vi "Configure DO Alarm.vi"(0 "VISA resource name":refnum<visa-resource-name>, 1 "Operation (0: And)":i32(ring) items=["And", "Or", "Reflash"], 2 "Hold / Non-Hold (Non-Hold)":bool, 3 "Operation When ACK (Normal)":u16(ring) items=["Normal", "Reset"], 5 "Channel Number (0001)":string="0001", 7 "Span And Energize":T1={"Span Lower Limit (0)"=0, "Span Upper Limit (1)"=1, "Unit (\"\")"="", "Output (De-Energize) "=FALSE} {"Span Upper Limit (1)" min=1 max=32; "Span Lower Limit (0)" min=1 max=32}, 9 "Reflash Time (500ms)":i32(ring) items=["500ms", "1s", "2s"], 11 "error in (no error)":errorcluster) -> (4 "VISA resource name out":refnum<visa-resource-name>, 6 "Channel Number":string, 15 "error out":errorcluster)   [LabVIEW 2020, in "Yokogawa GX Series.lvlib"]
doc: "Sets the DO alarm output related settings.\n\nCommand: SRangeDO"
uses:
  <instrlib>/Yokogawa GX Series/Yokogawa GX Series.lvlib
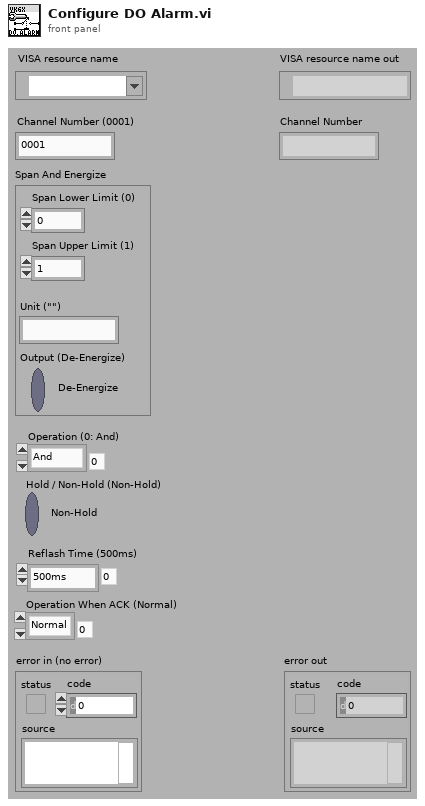
[diagram p1: front panel]
types:
  T1 = cluster{"Span Lower Limit (0)":i32, "Span Upper Limit (1)":i32, "Unit (\"\")":string, "Output (De-Energize) ":bool}
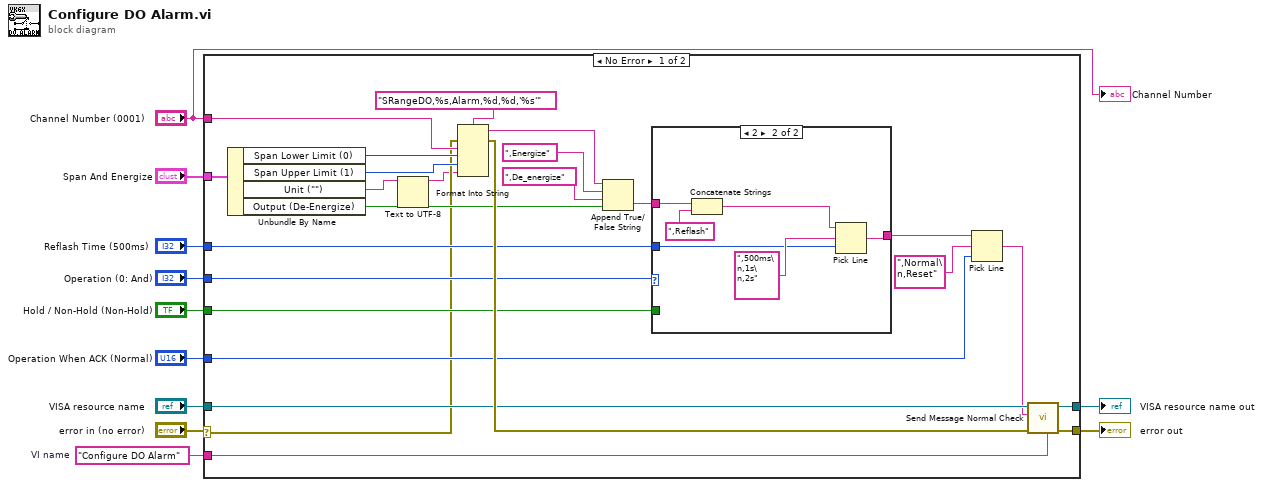
[diagram p0: block diagram]
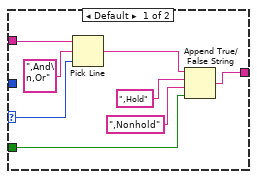
[diagram p2: hidden frame]
diagram:
  w1 = "Configure DO Alarm"  # VI name
  n1 = case shown="No Error" "error in (no error)" {
    selector: "error in (no error)" -> [w15 w51]
    tunnel: [w36 w52] -> w11
    tunnel: [w35 w51] -> w10
    tunnel: "VISA resource name" -> [w28 w52]
    tunnel: "Span And Energize" -> [w27 _]
    tunnel: "Hold / Non-Hold (Non-Hold)" -> [w22 _]
    tunnel: "Operation When ACK (Normal)" -> [w20 _]
    tunnel: "Operation (0: And)" -> [w18 _]
    tunnel: "Reflash Time (500ms)" -> [w17 _]
    tunnel: "Channel Number (0001)" -> [w16 _]
    tunnel: w1 -> [w14 _]
    frame No Error {
      n2 = Unbundle By Name(w27) -> ("Span Lower Limit (0)"=w26:i32, "Span Upper Limit (1)"=w25:i32, "Unit (\"\")"=w13:string, "Output (De-Energize)"=w24:bool)
      n3 = Text to UTF-8(11:w13) -> (3:w12:string)  [unwired: 2 in, 1 out]
      n4 = Format Into String(format string="SRangeDO,%s,Alarm,%d,%d,'%s'" ("形式文字列"), error in=w15, w16, w26, w25, w12) -> (resulting string=w31:string, error out=w29:errorcluster)  [unwired: 1 in]
      n5 = Append True/False String(1:w24, 2:",De_energize", 3:",Energize", 4:w31) -> (0:w30:string)
      n6 = case shown="2" w18 {
        selector: w18 -> [w38 _]
        tunnel: w30 -> [w42 w50]
        tunnel: w22 -> [w40 _]
        tunnel: [w39 w46] -> w21
        tunnel: w17 -> [_ w45]
        frame Default {
          n7 = Pick Line(string ("")=w42, multi-line string=",And\n,Or", line index=w38) -> (output string=w37:string)
          n8 = Append True/False String(1:w40, 2:",Nonhold", 3:",Hold", 4:w37) -> (0:w39:string)
        }
        frame 2 {
          n9 = Concatenate Strings(w50, ",Reflash") -> (w48:string)
          n10 = Pick Line(string ("")=w48, multi-line string=",500ms\n,1s\n,2s", line index=w45) -> (output string=w46:string)
        }
      }
      n11 = Pick Line(string ("")=w21, multi-line string=",Normal\n,Reset", line index=w20) -> (output string=w19:string)
      n12 = call <instrlib>:"Send Message Normal Check.vi"("Source (\"\")"=w14, "error in (no error)"=w29, "Send Message (\"\")"=w19, "VISA resource name"=w28) -> ("error out"=w35:errorcluster, "VISA resource name out"=w36:refnum<visa-resource-name>)  [unwired: 1 in, 5 out]
    }
    frame Error {
    }
  }
  "error out" <- w10
  "VISA resource name out" <- w11
  "Channel Number" <- "Channel Number (0001)"
